vi "plot_add_weather.vi"(5 "Input Points":dbl[](array[numeric])=[0.0, 0.0, 0.0], 9 "Input Arrays":dbl[][](array[numeric])=[[1.0, 4.0, 7.0], [2.0, 5.0, 8.0], [3.0, 6.0, 9.0]]) -> (10 "Output Arrays":dbl[][](array[numeric]), 13 "Timestamps":dbl[](array[numeric]))   [LabVIEW 2018]
doc: "Adds the datapoints for Timestamp, Rain Rate, and Accumulation to their corresponding plot arrays."
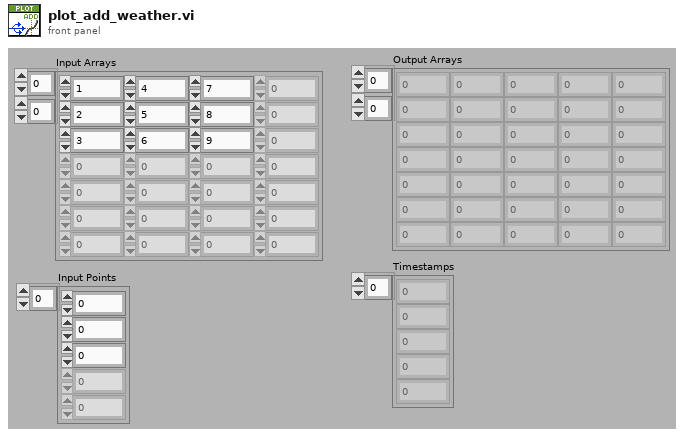
[diagram p1: front panel]
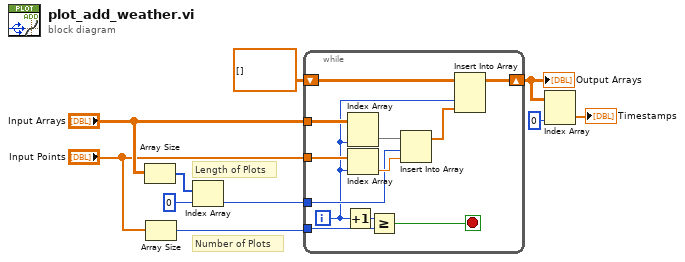
[diagram p0: block diagram]
diagram:
  # "Number of Plots"
  # "Length of Plots"
  n1 = Array Size(array="Input Arrays") -> (size(s)=w10:i32[])
  n2 = Array Size(array="Input Points") -> (size(s)=w2:i32)
  n3 = Index Array(array=w10, index=0) -> (element=w9:i32)
  n4 = while {
    tunnel: w2 -> [w14]
    tunnel: w9 -> [w15]
    tunnel: "Input Arrays" -> [w22]
    tunnel: "Input Points" -> [w21]
    shift-right: [w20] -> w5
    shift-left: dbl[][] [] ("Plot Arrays") -> [w18]
    i -> [w11]
    stop <- w13 stop-if-true
    n5 = Increment(x=w11) -> (x+1=w12:i32)
    n6 = Index Array(array=w22, index (col)=w11) -> (element=w17:dbl[])  [unwired: 1 in]
    n7 = Index Array(array=w21, index=w11) -> (element=w16:dbl)
    n8 = Greater Or Equal?(x=w12, y=w14) -> (x >= y?=w13:bool)
    n9 = Insert Into Array(array=w17, index=w15, new element=w16) -> (w19:dbl[])
    n10 = Insert Into Array(array=w18, index (col)=w11, new element=w19) -> (w20:dbl[][])  [unwired: 1 in]
  }
  "Output Arrays" <- w5
  n11 = Index Array(array=w5, index (col)=0 ("disabled index (col)")) -> (element=→"Timestamps":dbl[])  [unwired: 1 in]
